vi "Hitrap_DiagnosticBox.constructor.vi"(0 "name":string, 2 "data in":string, 5 "error in (no error)":errorcluster) -> (14 "i ref out":refnum<vi>, 16 "data out":string, 19 "error out":errorcluster)   [LabVIEW 2014, in "Hitrap_DiagnosticBox.lvlib"]
doc: "This is the constructor of a class.\n\nLicense Agreement for this software:\n\nCopyright (C)\nGesellschaft für Schwerionenforschung, GSI\nPlanckstr. 1\n64291 Darmstadt\nGermany\n\nContact: D.Beck@gsi.de \n\nThis program is free software; you can redistribute it and/or modify it under the terms of the \nGNU General Public License as published by the Free Software Foundation; either version 2 of \nthe license, or (at your option) any later version.\n\nThis program is distributed in the hope that it will be useful, but WITHOUT ANY WARRANTY; \nwithout even the implied warranty of MERCHANTABILITY or FITNESS FOR A PARTICULAR PURPOSE. See the GNU General License for more details (http://www.gnu.org).\n\nGesellschaft für Schwerionenforschung, GSI\nPlanckstr. 1, 64291 Darmstadt, Germany\nFor all questions and ideas contact: M.Richter@gsi.de, H.Brand@gsi.de or D.Beck@gsi.de.\nLast update: 16-JUN-2004"
uses:
  Hitrap_DiagnosticBox.lvlib
  CSCore/CSSystem/CSSystemLib/CSSystemLib.lvlib
  CSMotion/NanotecSMCPD/NanotecSMCPD.lvlib
  CSCore/CSObj/CSObj.lvlib
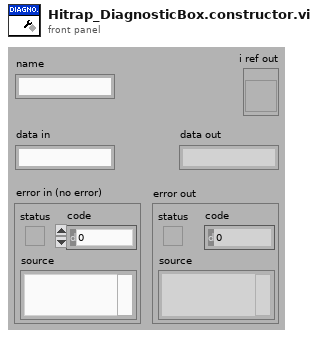
[diagram p1: front panel]
types:
  T1 = enum16{"SetAttribute", "GetAttribute", "CreateAttribute", "DestroyAttribute", "DestroyAllAtributes"}
  T2 = typedef "CSObj.lvlib/CSObj.i attribute.ctl" = cluster{"VI Refnum":refnum<vi>, "Front Panel Ref":refnum<vi>, "semaphore":T3, "date of birth":dbl, "ageID":i32, "systemID":i32, "classID":i32, "conditionID":i32, "DefaultPanelType":u16}
  T3 = typedef "Semaphore RefNum" = refnum<k1>
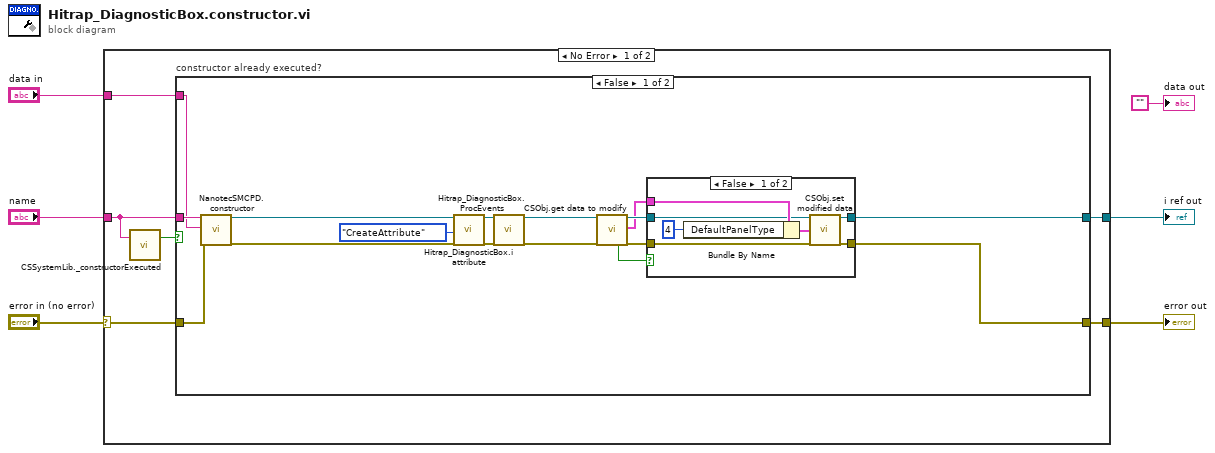
[diagram p0: block diagram]
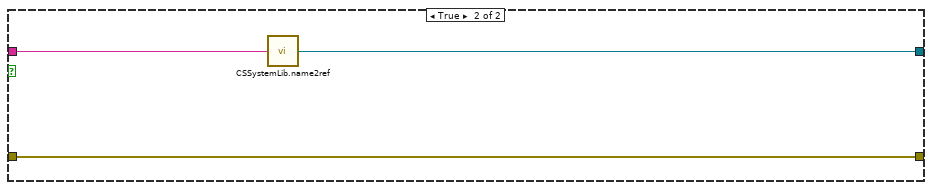
[diagram p3: hidden frame]
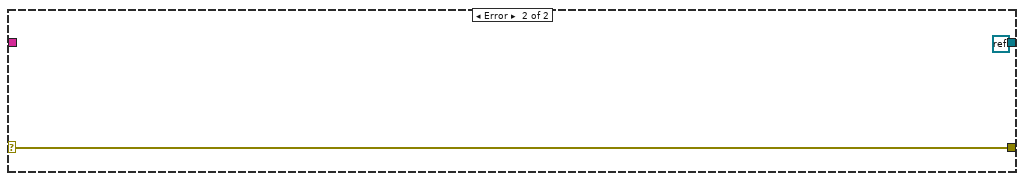
[diagram p4: hidden frame]
diagram:
  n1 = case shown="No Error" "error in (no error)" {
    selector: "error in (no error)" -> [w10 w41]
    tunnel: "name" -> [w9 _]
    tunnel: [w12 refnum<k0> refnum] -> w5
    tunnel: [w11 w41] -> w4
    tunnel: "data in" -> [w7 _]
    frame No Error {
      n2 = call "CSSystemLib._constructorExecuted.vi"("name"=w9) -> ("constructor executed?"=w8:bool)  [unwired: 18 in]
      n3 = case "constructor already executed?" shown="False" w8 {
        tunnel: w9 -> [w27 w40]
        tunnel: [w17 w39] -> w12
        tunnel: [w15 w38] -> w11
        tunnel: w10 -> [w24 w38]
        tunnel: w7 -> [w23 _]
        frame False {
          n4 = call "NanotecSMCPD.constructor.vi"("name"=w27, "data in"=w23, "error in (no error)"=w24) -> ("i ref out"=w14:refnum<vi>, "error out"=w13:errorcluster)  [unwired: 14 in, 1 out]
          n5 = call "Hitrap_DiagnosticBox.i attribute.vi"("VI Refnum"=w14, "Action"=T1."CreateAttribute", "error in (no error)"=w13) -> ("VI Refnum out"=w26:refnum<vi>, "error out"=w25:errorcluster)  [unwired: 14 in, 1 out]
          n6 = call "Hitrap_DiagnosticBox.ProcEvents.vi"("i ref in"=w26, "error in (no error)"=w25) -> ("i ref out"=w18:refnum<vi>, "error out"=w16:errorcluster)  [unwired: 16 in]
          n7 = call "CSObj.get data to modify.vi"("i ref in"=w18, "error in (no error)"=w16) -> ("i ref out"=w21:refnum<vi>, "i attribute"=w19:T2, "timed out"=w22:bool, "error out"=w20:errorcluster)  [unwired: 14 in]
          n8 = case shown="False" w22 {
            tunnel: [w33 w37] -> w17
            tunnel: w21 -> [w34 w37]
            tunnel: [w31 w36] -> w15
            tunnel: w20 -> [w32 w36]
            tunnel: w19 -> [w35 _]
            frame False {
              n9 = Bundle By Name(cluster=w35, "DefaultPanelType"=u16 4) -> (w30:T2)
              n10 = call "CSObj.set modified data.vi"("i ref in"=w34, "i attribute"=w30, "error in (no error)"=w32) -> ("i ref out"=w33:refnum<vi>, "error out"=w31:errorcluster)  [unwired: 15 in]
            }
            frame True {
            }
          }
        }
        frame True {
          n11 = call "CSSystemLib.name2ref.vi"("name"=w40) -> ("obj refnum"=w39:refnum<vi>)
        }
      }
    }
    frame Error {
    }
  }
  "i ref out" <- w5
  "error out" <- w4
  "data out" <- ""
